vi "Shock&Dyanamics Laboratory - DROPBEAR_June2022_Rev3.vi"() -> ()   [LabVIEW 2019] (continued)
                      tunnel: [w777 _] -> w775
                      frame #0 {
                        n215 = property on="PF Condition 13" class="Bool (strict)"() -> (error out=w778:errorcluster, "Value"=w781:bool)  [unwired: 2 in, 1 out]
                        n216 = case shown="True" w781 {
                          tunnel: [T42."Disabled and Grayed Out" ("Disabled") T42."Enabled" ("Disabled")] -> w782
                          frame False {
                          }
                          frame True {
                          }
                        }
                        n217 = property on="PF Chassis 13" class="DigNum (strict)"(error in=w778, "DisabledEnum"=w782) -> (error out=w779:errorcluster)  [unwired: 1 in, 1 out]
                        n218 = property on="PF Card 13" class="DigNum (strict)"(error in=w779, "DisabledEnum"=w782) -> (error out=w780:errorcluster)  [unwired: 1 in, 1 out]
                        n219 = property on="PF Channel 13" class="DigNum (strict)"(error in=w780, "DisabledEnum"=w782) -> (error out=w777:errorcluster)  [unwired: 1 in, 1 out]
                      }
                      frame #1 {
                        n220 = property on="Signal Type 13" class="Enum (strict)"() -> (error out=w788:errorcluster, "Value"=w787:T8)  [unwired: 2 in, 1 out]
                        n221 = case shown="\"Voltage\", Default" w787 {
                          tunnel: [T42."Enabled" ("Disabled") T42."Disabled and Grayed Out" ("Disabled")] -> w786
                          frame "Strain" {
                          }
                          frame "Voltage", Default {
                          }
                        }
                        n222 = property on="SG Pair 13" class="Bool (strict)"(error in=w788, "DisabledEnum"=w786) -> (error out=w785:errorcluster)  [unwired: 1 in, 1 out]
                        n223 = property on="SG Pair Ch 13" class="Enum (strict)"(error in=w785, "DisabledEnum"=w786) -> ()  [unwired: 1 in, 2 out]
                      }
                    }
                  }
                }
                n224 = case shown="True" w222 {
                  tunnel: [w727 T42."Enabled" ("Disabled")] -> w229
                  tunnel: [w728 w731] -> w227
                  frame False {
                    w727 = T42."Disabled and Grayed Out" ("Disabled")
                    n225 = property on="SG Pair 15" class="Bool (strict)"("DisabledEnum"=w727) -> (error out=w726:errorcluster)  [unwired: 2 in, 1 out]
                    n226 = property on="SG Pair Ch 15" class="Enum (strict)"(error in=w726, "DisabledEnum"=w727) -> (error out=w725:errorcluster)  [unwired: 1 in, 1 out]
                    n227 = property on="PF Chassis 15" class="DigNum (strict)"(error in=w725, "DisabledEnum"=w727) -> (error out=w730:errorcluster)  [unwired: 1 in, 1 out]
                    n228 = property on="PF Card 15" class="DigNum (strict)"(error in=w730, "DisabledEnum"=w727) -> (error out=w729:errorcluster)  [unwired: 1 in, 1 out]
                    n229 = property on="PF Channel 15" class="DigNum (strict)"(error in=w729, "DisabledEnum"=w727) -> (error out=w728:errorcluster)  [unwired: 1 in, 1 out]
                  }
                  frame True {
                    n230 = stacked-sequence {
                      tunnel: [w733 _] -> w731
                      frame #0 {
                        n231 = property on="PF Condition 15" class="Bool (strict)"() -> (error out=w734:errorcluster, "Value"=w737:bool)  [unwired: 2 in, 1 out]
                        n232 = case shown="True" w737 {
                          tunnel: [T42."Disabled and Grayed Out" ("Disabled") T42."Enabled" ("Disabled")] -> w738
                          frame False {
                          }
                          frame True {
                          }
                        }
                        n233 = property on="PF Chassis 15" class="DigNum (strict)"(error in=w734, "DisabledEnum"=w738) -> (error out=w735:errorcluster)  [unwired: 1 in, 1 out]
                        n234 = property on="PF Card 15" class="DigNum (strict)"(error in=w735, "DisabledEnum"=w738) -> (error out=w736:errorcluster)  [unwired: 1 in, 1 out]
                        n235 = property on="PF Channel 15" class="DigNum (strict)"(error in=w736, "DisabledEnum"=w738) -> (error out=w733:errorcluster)  [unwired: 1 in, 1 out]
                      }
                      frame #1 {
                        n236 = property on="Signal Type 15" class="Enum (strict)"() -> (error out=w744:errorcluster, "Value"=w743:T8)  [unwired: 2 in, 1 out]
                        n237 = case shown="\"Strain\"" w743 {
                          tunnel: [T42."Enabled" ("Disabled") T42."Disabled and Grayed Out" ("Disabled")] -> w742
                          frame "Strain" {
                          }
                          frame "Voltage", Default {
                          }
                        }
                        n238 = property on="SG Pair 15" class="Bool (strict)"(error in=w744, "DisabledEnum"=w742) -> (error out=w741:errorcluster)  [unwired: 1 in, 1 out]
                        n239 = property on="SG Pair Ch 15" class="Enum (strict)"(error in=w741, "DisabledEnum"=w742) -> ()  [unwired: 1 in, 2 out]
                      }
                    }
                  }
                }
                n240 = case shown="True" w302 {
                  tunnel: [w903 T42."Enabled" ("Disabled")] -> w306
                  tunnel: [w904 w907] -> w304
                  frame False {
                    w903 = T42."Disabled and Grayed Out" ("Disabled")
                    n241 = property on="SG Pair 7" class="Bool (strict)"("DisabledEnum"=w903) -> (error out=w902:errorcluster)  [unwired: 2 in, 1 out]
                    n242 = property on="SG Pair Ch 7" class="Enum (strict)"(error in=w902, "DisabledEnum"=w903) -> (error out=w901:errorcluster)  [unwired: 1 in, 1 out]
                    n243 = property on="PF Chassis 7" class="DigNum (strict)"(error in=w901, "DisabledEnum"=w903) -> (error out=w906:errorcluster)  [unwired: 1 in, 1 out]
                    n244 = property on="PF Card 7" class="DigNum (strict)"(error in=w906, "DisabledEnum"=w903) -> (error out=w905:errorcluster)  [unwired: 1 in, 1 out]
                    n245 = property on="PF Channel 7" class="DigNum (strict)"(error in=w905, "DisabledEnum"=w903) -> (error out=w904:errorcluster)  [unwired: 1 in, 1 out]
                  }
                  frame True {
                    n246 = stacked-sequence {
                      tunnel: [w909 _] -> w907
                      frame #0 {
                        n247 = property on="PF Condition 7" class="Bool (strict)"() -> (error out=w910:errorcluster, "Value"=w913:bool)  [unwired: 2 in, 1 out]
                        n248 = case shown="True" w913 {
                          tunnel: [T42."Disabled and Grayed Out" ("Disabled") T42."Enabled" ("Disabled")] -> w914
                          frame False {
                          }
                          frame True {
                          }
                        }
                        n249 = property on="PF Chassis 7" class="DigNum (strict)"(error in=w910, "DisabledEnum"=w914) -> (error out=w911:errorcluster)  [unwired: 1 in, 1 out]
                        n250 = property on="PF Card 7" class="DigNum (strict)"(error in=w911, "DisabledEnum"=w914) -> (error out=w912:errorcluster)  [unwired: 1 in, 1 out]
                        n251 = property on="PF Channel 7" class="DigNum (strict)"(error in=w912, "DisabledEnum"=w914) -> (error out=w909:errorcluster)  [unwired: 1 in, 1 out]
                      }
                      frame #1 {
                        n252 = property on="Signal Type 7" class="Enum (strict)"() -> (error out=w920:errorcluster, "Value"=w919:T8)  [unwired: 2 in, 1 out]
                        n253 = case shown="\"Voltage\", Default" w919 {
                          tunnel: [T42."Enabled" ("Disabled") T42."Disabled and Grayed Out" ("Disabled")] -> w918
                          frame "Strain" {
                          }
                          frame "Voltage", Default {
                          }
                        }
                        n254 = property on="SG Pair 7" class="Bool (strict)"(error in=w920, "DisabledEnum"=w918) -> (error out=w917:errorcluster)  [unwired: 1 in, 1 out]
                        n255 = property on="SG Pair Ch 7" class="Enum (strict)"(error in=w917, "DisabledEnum"=w918) -> ()  [unwired: 1 in, 2 out]
                      }
                    }
                  }
                }
                n256 = case shown="False" w226 {
                  tunnel: [w815 T42."Enabled" ("Disabled")] -> w265
                  tunnel: [w816 w819] -> w263
                  frame False {
                    w815 = T42."Disabled and Grayed Out" ("Disabled")
                    n257 = property on="SG Pair 11" class="Bool (strict)"("DisabledEnum"=w815) -> (error out=w814:errorcluster)  [unwired: 2 in, 1 out]
                    n258 = property on="SG Pair Ch 11" class="Enum (strict)"(error in=w814, "DisabledEnum"=w815) -> (error out=w813:errorcluster)  [unwired: 1 in, 1 out]
                    n259 = property on="PF Chassis 11" class="DigNum (strict)"(error in=w813, "DisabledEnum"=w815) -> (error out=w818:errorcluster)  [unwired: 1 in, 1 out]
                    n260 = property on="PF Card 11" class="DigNum (strict)"(error in=w818, "DisabledEnum"=w815) -> (error out=w817:errorcluster)  [unwired: 1 in, 1 out]
                    n261 = property on="PF Channel 11" class="DigNum (strict)"(error in=w817, "DisabledEnum"=w815) -> (error out=w816:errorcluster)  [unwired: 1 in, 1 out]
                  }
                  frame True {
                    n262 = stacked-sequence {
                      tunnel: [w821 _] -> w819
                      frame #0 {
                        n263 = property on="PF Condition 11" class="Bool (strict)"() -> (error out=w822:errorcluster, "Value"=w825:bool)  [unwired: 2 in, 1 out]
                        n264 = case shown="True" w825 {
                          tunnel: [T42."Disabled and Grayed Out" ("Disabled") T42."Enabled" ("Disabled")] -> w826
                          frame False {
                          }
                          frame True {
                          }
                        }
                        n265 = property on="PF Chassis 11" class="DigNum (strict)"(error in=w822, "DisabledEnum"=w826) -> (error out=w823:errorcluster)  [unwired: 1 in, 1 out]
                        n266 = property on="PF Card 11" class="DigNum (strict)"(error in=w823, "DisabledEnum"=w826) -> (error out=w824:errorcluster)  [unwired: 1 in, 1 out]
                        n267 = property on="PF Channel 11" class="DigNum (strict)"(error in=w824, "DisabledEnum"=w826) -> (error out=w821:errorcluster)  [unwired: 1 in, 1 out]
                      }
                      frame #1 {
                        n268 = property on="Signal Type 11" class="Enum (strict)"() -> (error out=w832:errorcluster, "Value"=w831:T8)  [unwired: 2 in, 1 out]
                        n269 = case shown="\"Voltage\", Default" w831 {
                          tunnel: [T42."Enabled" ("Disabled") T42."Disabled and Grayed Out" ("Disabled")] -> w830
                          frame "Strain" {
                          }
                          frame "Voltage", Default {
                          }
                        }
                        n270 = property on="SG Pair 11" class="Bool (strict)"(error in=w832, "DisabledEnum"=w830) -> (error out=w829:errorcluster)  [unwired: 1 in, 1 out]
                        n271 = property on="SG Pair Ch 11" class="Enum (strict)"(error in=w829, "DisabledEnum"=w830) -> ()  [unwired: 1 in, 2 out]
                      }
                    }
                  }
                }
                n272 = case shown="False" w223 {
                  tunnel: [w749 T42."Enabled" ("Disabled")] -> w238
                  tunnel: [w750 w753] -> w236
                  frame False {
                    w749 = T42."Disabled and Grayed Out" ("Disabled")
                    n273 = property on="SG Pair 14" class="Bool (strict)"("DisabledEnum"=w749) -> (error out=w748:errorcluster)  [unwired: 2 in, 1 out]
                    n274 = property on="SG Pair Ch 14" class="Enum (strict)"(error in=w748, "DisabledEnum"=w749) -> (error out=w747:errorcluster)  [unwired: 1 in, 1 out]
                    n275 = property on="PF Chassis 14" class="DigNum (strict)"(error in=w747, "DisabledEnum"=w749) -> (error out=w752:errorcluster)  [unwired: 1 in, 1 out]
                    n276 = property on="PF Card 14" class="DigNum (strict)"(error in=w752, "DisabledEnum"=w749) -> (error out=w751:errorcluster)  [unwired: 1 in, 1 out]
                    n277 = property on="PF Channel 14" class="DigNum (strict)"(error in=w751, "DisabledEnum"=w749) -> (error out=w750:errorcluster)  [unwired: 1 in, 1 out]
                  }
                  frame True {
                    n278 = stacked-sequence {
                      tunnel: [w755 _] -> w753
                      frame #0 {
                        n279 = property on="PF Condition 14" class="Bool (strict)"() -> (error out=w756:errorcluster, "Value"=w759:bool)  [unwired: 2 in, 1 out]
                        n280 = case shown="True" w759 {
                          tunnel: [T42."Disabled and Grayed Out" ("Disabled") T42."Enabled" ("Disabled")] -> w760
                          frame False {
                          }
                          frame True {
                          }
                        }
                        n281 = property on="PF Chassis 14" class="DigNum (strict)"(error in=w756, "DisabledEnum"=w760) -> (error out=w757:errorcluster)  [unwired: 1 in, 1 out]
                        n282 = property on="PF Card 14" class="DigNum (strict)"(error in=w757, "DisabledEnum"=w760) -> (error out=w758:errorcluster)  [unwired: 1 in, 1 out]
                        n283 = property on="PF Channel 14" class="DigNum (strict)"(error in=w758, "DisabledEnum"=w760) -> (error out=w755:errorcluster)  [unwired: 1 in, 1 out]
                      }
                      frame #1 {
                        n284 = property on="Signal Type 14" class="Enum (strict)"() -> (error out=w766:errorcluster, "Value"=w765:T8)  [unwired: 2 in, 1 out]
                        n285 = case shown="\"Voltage\", Default" w765 {
                          tunnel: [T42."Enabled" ("Disabled") T42."Disabled and Grayed Out" ("Disabled")] -> w764
                          frame "Strain" {
                          }
                          frame "Voltage", Default {
                          }
                        }
                        n286 = property on="SG Pair 14" class="Bool (strict)"(error in=w766, "DisabledEnum"=w764) -> (error out=w763:errorcluster)  [unwired: 1 in, 1 out]
                        n287 = property on="SG Pair Ch 14" class="Enum (strict)"(error in=w763, "DisabledEnum"=w764) -> ()  [unwired: 1 in, 2 out]
                      }
                    }
                  }
                }
                n288 = case shown="False" w214 {
                  tunnel: [w705 T42."Enabled" ("Disabled")] -> w197
                  tunnel: [w706 w709] -> w198
                  frame False {
                    w705 = T42."Disabled and Grayed Out" ("Disabled")
                    n289 = property on="SG Pair 16" class="Bool (strict)"("DisabledEnum"=w705) -> (error out=w704:errorcluster)  [unwired: 2 in, 1 out]
                    n290 = property on="SG Pair Ch 16" class="Enum (strict)"(error in=w704, "DisabledEnum"=w705) -> (error out=w703:errorcluster)  [unwired: 1 in, 1 out]
                    n291 = property on="PF Chassis 16" class="DigNum (strict)"(error in=w703, "DisabledEnum"=w705) -> (error out=w708:errorcluster)  [unwired: 1 in, 1 out]
                    n292 = property on="PF Card 16" class="DigNum (strict)"(error in=w708, "DisabledEnum"=w705) -> (error out=w707:errorcluster)  [unwired: 1 in, 1 out]
                    n293 = property on="PF Channel 16" class="DigNum (strict)"(error in=w707, "DisabledEnum"=w705) -> (error out=w706:errorcluster)  [unwired: 1 in, 1 out]
                  }
                  frame True {
                    n294 = stacked-sequence {
                      tunnel: [w712 _] -> w709
                      frame #0 {
                        n295 = property on="PF Condition 16" class="Bool (strict)"() -> (error out=w713:errorcluster, "Value"=w716:bool)  [unwired: 2 in, 1 out]
                        n296 = case shown="True" w716 {
                          tunnel: [T42."Disabled and Grayed Out" ("Disabled") T42."Enabled" ("Disabled")] -> w711
                          frame False {
                          }
                          frame True {
                          }
                        }
                        n297 = property on="PF Chassis 16" class="DigNum (strict)"(error in=w713, "DisabledEnum"=w711) -> (error out=w714:errorcluster)  [unwired: 1 in, 1 out]
                        n298 = property on="PF Card 16" class="DigNum (strict)"(error in=w714, "DisabledEnum"=w711) -> (error out=w715:errorcluster)  [unwired: 1 in, 1 out]
                        n299 = property on="PF Channel 16" class="DigNum (strict)"(error in=w715, "DisabledEnum"=w711) -> (error out=w712:errorcluster)  [unwired: 1 in, 1 out]
                      }
                      frame #1 {
                        n300 = property on="Signal Type 16" class="Enum (strict)"() -> (error out=w722:errorcluster, "Value"=w721:T8)  [unwired: 2 in, 1 out]
                        n301 = case shown="\"Strain\"" w721 {
                          tunnel: [T42."Enabled" ("Disabled") T42."Disabled and Grayed Out" ("Disabled")] -> w720
                          frame "Strain" {
                          }
                          frame "Voltage", Default {
                          }
                        }
                        n302 = property on="SG Pair 16" class="Bool (strict)"(error in=w722, "DisabledEnum"=w720) -> (error out=w719:errorcluster)  [unwired: 1 in, 1 out]
                        n303 = property on="SG Pair Ch 16" class="Enum (strict)"(error in=w719, "DisabledEnum"=w720) -> ()  [unwired: 1 in, 2 out]
                      }
                    }
                  }
                }
                n304 = case shown="False" w274 {
                  tunnel: [w881 T42."Enabled" ("Disabled")] -> w295
                  tunnel: [w882 w885] -> w293
                  frame False {
                    w881 = T42."Disabled and Grayed Out" ("Disabled")
                    n305 = property on="SG Pair 8" class="Bool (strict)"("DisabledEnum"=w881) -> (error out=w880:errorcluster)  [unwired: 2 in, 1 out]
                    n306 = property on="SG Pair Ch 8" class="Enum (strict)"(error in=w880, "DisabledEnum"=w881) -> (error out=w879:errorcluster)  [unwired: 1 in, 1 out]
                    n307 = property on="PF Chassis 8" class="DigNum (strict)"(error in=w879, "DisabledEnum"=w881) -> (error out=w884:errorcluster)  [unwired: 1 in, 1 out]
                    n308 = property on="PF Card 8" class="DigNum (strict)"(error in=w884, "DisabledEnum"=w881) -> (error out=w883:errorcluster)  [unwired: 1 in, 1 out]
                    n309 = property on="PF Channel 8" class="DigNum (strict)"(error in=w883, "DisabledEnum"=w881) -> (error out=w882:errorcluster)  [unwired: 1 in, 1 out]
                  }
                  frame True {
                    n310 = stacked-sequence {
                      tunnel: [w887 _] -> w885
                      frame #0 {
                        n311 = property on="PF Condition 8" class="Bool (strict)"() -> (error out=w888:errorcluster, "Value"=w891:bool)  [unwired: 2 in, 1 out]
                        n312 = case shown="True" w891 {
                          tunnel: [T42."Disabled and Grayed Out" ("Disabled") T42."Enabled" ("Disabled")] -> w892
                          frame False {
                          }
                          frame True {
                          }
                        }
                        n313 = property on="PF Chassis 8" class="DigNum (strict)"(error in=w888, "DisabledEnum"=w892) -> (error out=w889:errorcluster)  [unwired: 1 in, 1 out]
                        n314 = property on="PF Card 8" class="DigNum (strict)"(error in=w889, "DisabledEnum"=w892) -> (error out=w890:errorcluster)  [unwired: 1 in, 1 out]
                        n315 = property on="PF Channel 8" class="DigNum (strict)"(error in=w890, "DisabledEnum"=w892) -> (error out=w887:errorcluster)  [unwired: 1 in, 1 out]
                      }
                      frame #1 {
                        n316 = property on="Signal Type 8" class="Enum (strict)"() -> (error out=w898:errorcluster, "Value"=w897:T8)  [unwired: 2 in, 1 out]
                        n317 = case shown="\"Voltage\", Default" w897 {
                          tunnel: [T42."Enabled" ("Disabled") T42."Disabled and Grayed Out" ("Disabled")] -> w896
                          frame "Strain" {
                          }
                          frame "Voltage", Default {
                          }
                        }
                        n318 = property on="SG Pair 8" class="Bool (strict)"(error in=w898, "DisabledEnum"=w896) -> (error out=w895:errorcluster)  [unwired: 1 in, 1 out]
                        n319 = property on="SG Pair Ch 8" class="Enum (strict)"(error in=w895, "DisabledEnum"=w896) -> ()  [unwired: 1 in, 2 out]
                      }
                    }
                  }
                }
                n320 = case shown="False" w273 {
                  tunnel: [w859 T42."Enabled" ("Disabled")] -> w286
                  tunnel: [w860 w863] -> w284
                  frame False {
                    w859 = T42."Disabled and Grayed Out" ("Disabled")
                    n321 = property on="SG Pair 9" class="Bool (strict)"("DisabledEnum"=w859) -> (error out=w858:errorcluster)  [unwired: 2 in, 1 out]
                    n322 = property on="SG Pair Ch 9" class="Enum (strict)"(error in=w858, "DisabledEnum"=w859) -> (error out=w857:errorcluster)  [unwired: 1 in, 1 out]
                    n323 = property on="PF Chassis 9" class="DigNum (strict)"(error in=w857, "DisabledEnum"=w859) -> (error out=w862:errorcluster)  [unwired: 1 in, 1 out]
                    n324 = property on="PF Card 9" class="DigNum (strict)"(error in=w862, "DisabledEnum"=w859) -> (error out=w861:errorcluster)  [unwired: 1 in, 1 out]
                    n325 = property on="PF Channel 9" class="DigNum (strict)"(error in=w861, "DisabledEnum"=w859) -> (error out=w860:errorcluster)  [unwired: 1 in, 1 out]
                  }
                  frame True {
                    n326 = stacked-sequence {
                      tunnel: [w865 _] -> w863
                      frame #0 {
                        n327 = property on="PF Condition 9" class="Bool (strict)"() -> (error out=w866:errorcluster, "Value"=w869:bool)  [unwired: 2 in, 1 out]
                        n328 = case shown="True" w869 {
                          tunnel: [T42."Disabled and Grayed Out" ("Disabled") T42."Enabled" ("Disabled")] -> w870
                          frame False {
                          }
                          frame True {
                          }
                        }
                        n329 = property on="PF Chassis 9" class="DigNum (strict)"(error in=w866, "DisabledEnum"=w870) -> (error out=w867:errorcluster)  [unwired: 1 in, 1 out]
                        n330 = property on="PF Card 9" class="DigNum (strict)"(error in=w867, "DisabledEnum"=w870) -> (error out=w868:errorcluster)  [unwired: 1 in, 1 out]
                        n331 = property on="PF Channel 9" class="DigNum (strict)"(error in=w868, "DisabledEnum"=w870) -> (error out=w865:errorcluster)  [unwired: 1 in, 1 out]
                      }
                      frame #1 {
                        n332 = property on="Signal Type 9" class="Enum (strict)"() -> (error out=w876:errorcluster, "Value"=w875:T8)  [unwired: 2 in, 1 out]
                        n333 = case shown="\"Voltage\", Default" w875 {
                          tunnel: [T42."Enabled" ("Disabled") T42."Disabled and Grayed Out" ("Disabled")] -> w874
                          frame "Strain" {
                          }
                          frame "Voltage", Default {
                          }
                        }
                        n334 = property on="SG Pair 9" class="Bool (strict)"(error in=w876, "DisabledEnum"=w874) -> (error out=w873:errorcluster)  [unwired: 1 in, 1 out]
                        n335 = property on="SG Pair Ch 9" class="Enum (strict)"(error in=w873, "DisabledEnum"=w874) -> ()  [unwired: 1 in, 2 out]
                      }
                    }
                  }
                }
                n336 = case shown="False" w272 {
                  tunnel: [w837 T42."Enabled" ("Disabled")] -> w277
                  tunnel: [w838 w841] -> w275
                  frame False {
                    w837 = T42."Disabled and Grayed Out" ("Disabled")
                    n337 = property on="SG Pair 10" class="Bool (strict)"("DisabledEnum"=w837) -> (error out=w836:errorcluster)  [unwired: 2 in, 1 out]
                    n338 = property on="SG Pair Ch 10" class="Enum (strict)"(error in=w836, "DisabledEnum"=w837) -> (error out=w835:errorcluster)  [unwired: 1 in, 1 out]
                    n339 = property on="PF Chassis 10" class="DigNum (strict)"(error in=w835, "DisabledEnum"=w837) -> (error out=w840:errorcluster)  [unwired: 1 in, 1 out]
                    n340 = property on="PF Card 10" class="DigNum (strict)"(error in=w840, "DisabledEnum"=w837) -> (error out=w839:errorcluster)  [unwired: 1 in, 1 out]
                    n341 = property on="PF Channel 10" class="DigNum (strict)"(error in=w839, "DisabledEnum"=w837) -> (error out=w838:errorcluster)  [unwired: 1 in, 1 out]
                  }
                  frame True {
                    n342 = stacked-sequence {
                      tunnel: [w843 _] -> w841
                      frame #0 {
                        n343 = property on="PF Condition 10" class="Bool (strict)"() -> (error out=w844:errorcluster, "Value"=w847:bool)  [unwired: 2 in, 1 out]
                        n344 = case shown="True" w847 {
                          tunnel: [T42."Disabled and Grayed Out" ("Disabled") T42."Enabled" ("Disabled")] -> w848
                          frame False {
                          }
                          frame True {
                          }
                        }
                        n345 = property on="PF Chassis 10" class="DigNum (strict)"(error in=w844, "DisabledEnum"=w848) -> (error out=w845:errorcluster)  [unwired: 1 in, 1 out]
                        n346 = property on="PF Card 10" class="DigNum (strict)"(error in=w845, "DisabledEnum"=w848) -> (error out=w846:errorcluster)  [unwired: 1 in, 1 out]
                        n347 = property on="PF Channel 10" class="DigNum (strict)"(error in=w846, "DisabledEnum"=w848) -> (error out=w843:errorcluster)  [unwired: 1 in, 1 out]
                      }
                      frame #1 {
                        n348 = property on="Signal Type 10" class="Enum (strict)"() -> (error out=w854:errorcluster, "Value"=w853:T8)  [unwired: 2 in, 1 out]
                        n349 = case shown="\"Voltage\", Default" w853 {
                          tunnel: [T42."Enabled" ("Disabled") T42."Disabled and Grayed Out" ("Disabled")] -> w852
                          frame "Strain" {
                          }
                          frame "Voltage", Default {
                          }
                        }
                        n350 = property on="SG Pair 10" class="Bool (strict)"(error in=w854, "DisabledEnum"=w852) -> (error out=w851:errorcluster)  [unwired: 1 in, 1 out]
                        n351 = property on="SG Pair Ch 10" class="Enum (strict)"(error in=w851, "DisabledEnum"=w852) -> ()  [unwired: 1 in, 2 out]
                      }
                    }
                  }
                }
                n352 = case shown="True" w213 {
                  tunnel: [w683 T42."Enabled" ("Disabled")] -> w187
                  tunnel: [w686 w687] -> w195
                  frame False {
                    w683 = T42."Disabled and Grayed Out" ("Disabled")
                    n353 = property on="SG Pair 17" class="Bool (strict)"("DisabledEnum"=w683) -> (error out=w682:errorcluster)  [unwired: 2 in, 1 out]
                    n354 = property on="SG Pair Ch 17" class="Enum (strict)"(error in=w682, "DisabledEnum"=w683) -> (error out=w681:errorcluster)  [unwired: 1 in, 1 out]
                    n355 = property on="PF Chassis 17" class="DigNum (strict)"(error in=w681, "DisabledEnum"=w683) -> (error out=w684:errorcluster)  [unwired: 1 in, 1 out]
                    n356 = property on="PF Card 17" class="DigNum (strict)"(error in=w684, "DisabledEnum"=w683) -> (error out=w685:errorcluster)  [unwired: 1 in, 1 out]
                    n357 = property on="PF Channel 17" class="DigNum (strict)"(error in=w685, "DisabledEnum"=w683) -> (error out=w686:errorcluster)  [unwired: 1 in, 1 out]
                  }
                  frame True {
                    n358 = stacked-sequence {
                      tunnel: [w693 _] -> w687
                      frame #0 {
                        n359 = property on="PF Condition 17" class="Bool (strict)"() -> (error out=w690:errorcluster, "Value"=w694:bool)  [unwired: 2 in, 1 out]
                        n360 = case shown="True" w694 {
                          tunnel: [T42."Disabled and Grayed Out" ("Disabled") T42."Enabled" ("Disabled")] -> w689
                          frame False {
                          }
                          frame True {
                          }
                        }
                        n361 = property on="PF Chassis 17" class="DigNum (strict)"(error in=w690, "DisabledEnum"=w689) -> (error out=w691:errorcluster)  [unwired: 1 in, 1 out]
                        n362 = property on="PF Card 17" class="DigNum (strict)"(error in=w691, "DisabledEnum"=w689) -> (error out=w692:errorcluster)  [unwired: 1 in, 1 out]
                        n363 = property on="PF Channel 17" class="DigNum (strict)"(error in=w692, "DisabledEnum"=w689) -> (error out=w693:errorcluster)  [unwired: 1 in, 1 out]
                      }
                      frame #1 {
                        n364 = property on="Signal Type 17" class="Enum (strict)"() -> (error out=w699:errorcluster, "Value"=w700:T8)  [unwired: 2 in, 1 out]
                        n365 = case shown="\"Voltage\", Default" w700 {
                          tunnel: [T42."Enabled" ("Disabled") T42."Disabled and Grayed Out" ("Disabled")] -> w698
                          frame "Strain" {
                          }
                          frame "Voltage", Default {
                          }
                        }
                        n366 = property on="SG Pair 17" class="Bool (strict)"(error in=w699, "DisabledEnum"=w698) -> (error out=w697:errorcluster)  [unwired: 1 in, 1 out]
                        n367 = property on="SG Pair Ch 17" class="Enum (strict)"(error in=w697, "DisabledEnum"=w698) -> ()  [unwired: 1 in, 2 out]
                      }
                    }
                  }
                }
                n368 = case shown="False" w210 {
                  tunnel: [w617 T42."Enabled" ("Disabled")] -> w160
                  tunnel: [w618 w621] -> w168
                  frame False {
                    w617 = T42."Disabled and Grayed Out" ("Disabled")
                    n369 = property on="SG Pair 20" class="Bool (strict)"("DisabledEnum"=w617) -> (error out=w616:errorcluster)  [unwired: 2 in, 1 out]
                    n370 = property on="SG Pair Ch 20" class="Enum (strict)"(error in=w616, "DisabledEnum"=w617) -> (error out=w615:errorcluster)  [unwired: 1 in, 1 out]
                    n371 = property on="PF Chassis 20" class="DigNum (strict)"(error in=w615, "DisabledEnum"=w617) -> (error out=w620:errorcluster)  [unwired: 1 in, 1 out]
                    n372 = property on="PF Card 20" class="DigNum (strict)"(error in=w620, "DisabledEnum"=w617) -> (error out=w619:errorcluster)  [unwired: 1 in, 1 out]
                    n373 = property on="PF Channel 20" class="DigNum (strict)"(error in=w619, "DisabledEnum"=w617) -> (error out=w618:errorcluster)  [unwired: 1 in, 1 out]
                  }
                  frame True {
                    n374 = stacked-sequence {
                      tunnel: [w627 _] -> w621
                      frame #0 {
                        n375 = property on="PF Condition 20" class="Bool (strict)"() -> (error out=w624:errorcluster, "Value"=w628:bool)  [unwired: 2 in, 1 out]
                        n376 = case shown="True" w628 {
                          tunnel: [T42."Disabled and Grayed Out" ("Disabled") T42."Enabled" ("Disabled")] -> w623
                          frame False {
                          }
                          frame True {
                          }
                        }
                        n377 = property on="PF Chassis 20" class="DigNum (strict)"(error in=w624, "DisabledEnum"=w623) -> (error out=w625:errorcluster)  [unwired: 1 in, 1 out]
                        n378 = property on="PF Card 20" class="DigNum (strict)"(error in=w625, "DisabledEnum"=w623) -> (error out=w626:errorcluster)  [unwired: 1 in, 1 out]
                        n379 = property on="PF Channel 20" class="DigNum (strict)"(error in=w626, "DisabledEnum"=w623) -> (error out=w627:errorcluster)  [unwired: 1 in, 1 out]
                      }
                      frame #1 {
                        n380 = property on="Signal Type 20" class="Enum (strict)"() -> (error out=w634:errorcluster, "Value"=w633:T8)  [unwired: 2 in, 1 out]
                        n381 = case shown="\"Voltage\", Default" w633 {
                          tunnel: [T42."Enabled" ("Disabled") T42."Disabled and Grayed Out" ("Disabled")] -> w632
                          frame "Strain" {
                          }
                          frame "Voltage", Default {
                          }
                        }
                        n382 = property on="SG Pair 20" class="Bool (strict)"(error in=w634, "DisabledEnum"=w632) -> (error out=w631:errorcluster)  [unwired: 1 in, 1 out]
                        n383 = property on="SG Pair Ch 20" class="Enum (strict)"(error in=w631, "DisabledEnum"=w632) -> ()  [unwired: 1 in, 2 out]
                      }
                    }
                  }
                }
                n384 = case shown="False" w209 {
                  tunnel: [w595 T42."Enabled" ("Disabled")] -> w127
                  tunnel: [w596 w599] -> w159
                  frame False {
                    w595 = T42."Disabled and Grayed Out" ("Disabled")
                    n385 = property on="SG Pair 21" class="Bool (strict)"("DisabledEnum"=w595) -> (error out=w594:errorcluster)  [unwired: 2 in, 1 out]
                    n386 = property on="SG Pair Ch 21" class="Enum (strict)"(error in=w594, "DisabledEnum"=w595) -> (error out=w593:errorcluster)  [unwired: 1 in, 1 out]
                    n387 = property on="PF Chassis 21" class="DigNum (strict)"(error in=w593, "DisabledEnum"=w595) -> (error out=w598:errorcluster)  [unwired: 1 in, 1 out]
                    n388 = property on="PF Card 21" class="DigNum (strict)"(error in=w598, "DisabledEnum"=w595) -> (error out=w597:errorcluster)  [unwired: 1 in, 1 out]
                    n389 = property on="PF Channel 21" class="DigNum (strict)"(error in=w597, "DisabledEnum"=w595) -> (error out=w596:errorcluster)  [unwired: 1 in, 1 out]
                  }
                  frame True {
                    n390 = stacked-sequence {
                      tunnel: [w604 _] -> w599
                      frame #0 {
                        n391 = property on="PF Condition 21" class="Bool (strict)"() -> (error out=w601:errorcluster, "Value"=w606:bool)  [unwired: 2 in, 1 out]
                        n392 = case shown="True" w606 {
                          tunnel: [T42."Disabled and Grayed Out" ("Disabled") T42."Enabled" ("Disabled")] -> w605
                          frame False {
                          }
                          frame True {
                          }
                        }
                        n393 = property on="PF Chassis 21" class="DigNum (strict)"(error in=w601, "DisabledEnum"=w605) -> (error out=w602:errorcluster)  [unwired: 1 in, 1 out]
                        n394 = property on="PF Card 21" class="DigNum (strict)"(error in=w602, "DisabledEnum"=w605) -> (error out=w603:errorcluster)  [unwired: 1 in, 1 out]
                        n395 = property on="PF Channel 21" class="DigNum (strict)"(error in=w603, "DisabledEnum"=w605) -> (error out=w604:errorcluster)  [unwired: 1 in, 1 out]
                      }
                      frame #1 {
                        n396 = property on="Signal Type 21" class="Enum (strict)"() -> (error out=w611:errorcluster, "Value"=w612:T8)  [unwired: 2 in, 1 out]
                        n397 = case shown="\"Voltage\", Default" w612 {
                          tunnel: [T42."Enabled" ("Disabled") T42."Disabled and Grayed Out" ("Disabled")] -> w610
                          frame "Strain" {
                          }
                          frame "Voltage", Default {
                          }
                        }
                        n398 = property on="SG Pair 21" class="Bool (strict)"(error in=w611, "DisabledEnum"=w610) -> (error out=w609:errorcluster)  [unwired: 1 in, 1 out]
                        n399 = property on="SG Pair Ch 21" class="Enum (strict)"(error in=w609, "DisabledEnum"=w610) -> ()  [unwired: 1 in, 2 out]
                      }
                    }
                  }
                }
                n400 = case shown="False" w207 {
                  tunnel: [w551 T42."Enabled" ("Disabled")] -> w125
                  tunnel: [w554 w555] -> w143
                  frame False {
                    w551 = T42."Disabled and Grayed Out" ("Disabled")
                    n401 = property on="SG Pair 23" class="Bool (strict)"("DisabledEnum"=w551) -> (error out=w550:errorcluster)  [unwired: 2 in, 1 out]
                    n402 = property on="SG Pair Ch 23" class="Enum (strict)"(error in=w550, "DisabledEnum"=w551) -> (error out=w549:errorcluster)  [unwired: 1 in, 1 out]
                    n403 = property on="PF Chassis 23" class="DigNum (strict)"(error in=w549, "DisabledEnum"=w551) -> (error out=w552:errorcluster)  [unwired: 1 in, 1 out]
                    n404 = property on="PF Card 23" class="DigNum (strict)"(error in=w552, "DisabledEnum"=w551) -> (error out=w553:errorcluster)  [unwired: 1 in, 1 out]
                    n405 = property on="PF Channel 23" class="DigNum (strict)"(error in=w553, "DisabledEnum"=w551) -> (error out=w554:errorcluster)  [unwired: 1 in, 1 out]
                  }
                  frame True {
                    n406 = stacked-sequence {
                      tunnel: [w561 _] -> w555
                      frame #0 {
                        n407 = property on="PF Condition 23" class="Bool (strict)"() -> (error out=w558:errorcluster, "Value"=w562:bool)  [unwired: 2 in, 1 out]
                        n408 = case shown="True" w562 {
                          tunnel: [T42."Disabled and Grayed Out" ("Disabled") T42."Enabled" ("Disabled")] -> w557
                          frame False {
                          }
                          frame True {
                          }
                        }
                        n409 = property on="PF Chassis 23" class="DigNum (strict)"(error in=w558, "DisabledEnum"=w557) -> (error out=w559:errorcluster)  [unwired: 1 in, 1 out]
                        n410 = property on="PF Card 23" class="DigNum (strict)"(error in=w559, "DisabledEnum"=w557) -> (error out=w560:errorcluster)  [unwired: 1 in, 1 out]
                        n411 = property on="PF Channel 23" class="DigNum (strict)"(error in=w560, "DisabledEnum"=w557) -> (error out=w561:errorcluster)  [unwired: 1 in, 1 out]
                      }
                      frame #1 {
                        n412 = property on="Signal Type 23" class="Enum (strict)"() -> (error out=w567:errorcluster, "Value"=w568:T8)  [unwired: 2 in, 1 out]
                        n413 = case shown="\"Voltage\", Default" w568 {
                          tunnel: [T42."Enabled" ("Disabled") T42."Disabled and Grayed Out" ("Disabled")] -> w566
                          frame "Strain" {
                          }
                          frame "Voltage", Default {
                          }
                        }
                        n414 = property on="SG Pair 23" class="Bool (strict)"(error in=w567, "DisabledEnum"=w566) -> (error out=w565:errorcluster)  [unwired: 1 in, 1 out]
                        n415 = property on="SG Pair Ch 23" class="Enum (strict)"(error in=w565, "DisabledEnum"=w566) -> ()  [unwired: 1 in, 2 out]
                      }
                    }
                  }
                }
                n416 = case shown="True" w201 {
                  tunnel: [w419 T42."Enabled" ("Disabled")] -> w87
                  tunnel: [w422 w424] -> w79
                  frame False {
                    w419 = T42."Disabled and Grayed Out" ("Disabled")
                    n417 = property on="SG Pair 29" class="Bool (strict)"("DisabledEnum"=w419) -> (error out=w418:errorcluster)  [unwired: 2 in, 1 out]
                    n418 = property on="SG Pair Ch 29" class="Enum (strict)"(error in=w418, "DisabledEnum"=w419) -> (error out=w417:errorcluster)  [unwired: 1 in, 1 out]
                    n419 = property on="PF Chassis 29" class="DigNum (strict)"(error in=w417, "DisabledEnum"=w419) -> (error out=w420:errorcluster)  [unwired: 1 in, 1 out]
